vi "Process Imported Data.vi"(8 "error in (no error)":errorcluster, 10 "Raw File Data":string, 11 "State Data in":T1={"Raw File Data"="", "Deduplicated String Array"=[], "1-Entries"=[], "2-Entries"=[], "3-Entries"=[], "Bounds"={"M-Min"=0, "M-Max"=1023, "S-Min"=0, "S-Max"=1023}, "Matched ADC Values - Nearest"=[], "Match Entry Indices - Nearest"=[], "Filtered 1-Entries"=[], "Filtered 2-Entries"=[], "Filtered 3-Entries"=[], "Total Duration"=0.0, "Matched ADC Values - Largest"=[], "Match Entry Indices - Largest"=[]}) -> (0 "error out":errorcluster, 3 "State Data out":T1={"Raw File Data"="", "Deduplicated String Array"=[], "1-Entries"=[], "2-Entries"=[], "3-Entries"=[], "Bounds"={"M-Min"=0, "M-Max"=1023, "S-Min"=0, "S-Max"=1023}, "Matched ADC Values - Nearest"=[], "Match Entry Indices - Nearest"=[], "Filtered 1-Entries"=[], "Filtered 2-Entries"=[], "Filtered 3-Entries"=[], "Total Duration"=0.0, "Matched ADC Values - Largest"=[], "Match Entry Indices - Largest"=[]})   [LabVIEW 2019, in "Muon Data Post-Processing.lvlib"]
uses:
  Muon Data Post-Processing.lvlib
  State Data.ctl
  File Entry.ctl
  ADC Bounds.ctl
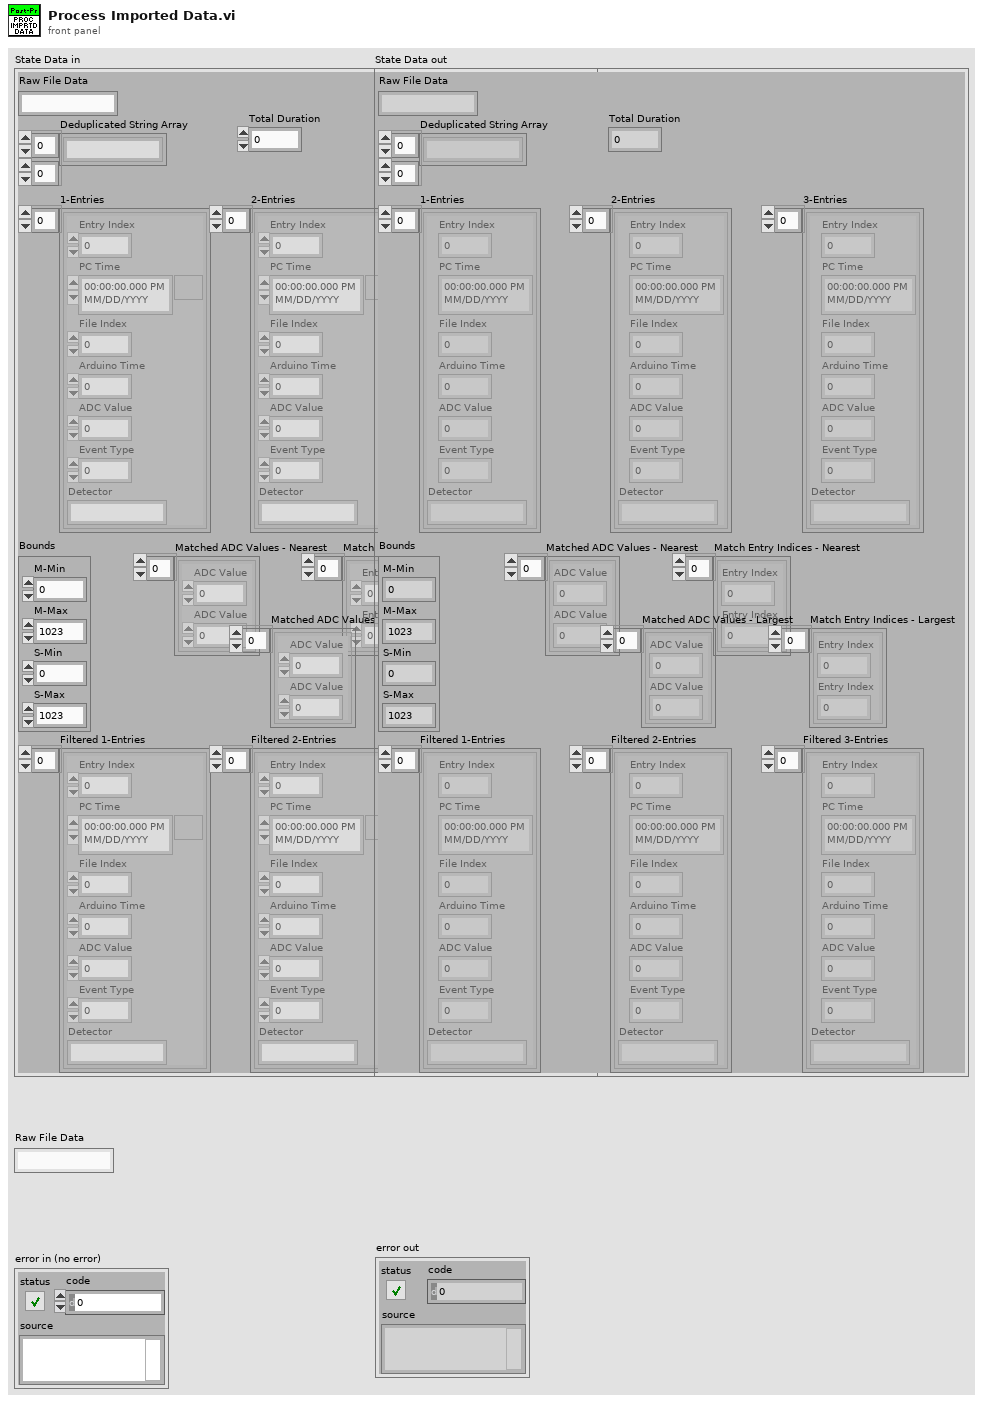
[diagram p1: front panel]
types:
  T1 = typedef "Muon Data Post-Processing.lvlib/State Data.ctl" = cluster{"Raw File Data":string, "Deduplicated String Array":string[][], "1-Entries":T2[], "2-Entries":T2[], "3-Entries":T2[], "Bounds":T3, "Matched ADC Values - Nearest":cluster{"ADC Value":i32, "ADC Value":i32}[], "Match Entry Indices - Nearest":cluster{"Entry Index":i32, "Entry Index":i32}[], "Filtered 1-Entries":T2[], "Filtered 2-Entries":T2[], "Filtered 3-Entries":T2[], "Total Duration":dbl, "Matched ADC Values - Largest":cluster{"ADC Value":i32, "ADC Value":i32}[], "Match Entry Indices - Largest":cluster{"Entry Index":i32, "Entry Index":i32}[]}
  T2 = typedef "Muon Data Post-Processing.lvlib/File Entry.ctl" = cluster{"Entry Index":i32, "PC Time":timestamp, "File Index":i32, "Arduino Time":i32, "ADC Value":i32, "Event Type":i32, "Detector":string}
  T3 = typedef "Muon Data Post-Processing.lvlib/ADC Bounds.ctl" = cluster{"M-Min":u16, "M-Max":u16, "S-Min":u16, "S-Max":u16}
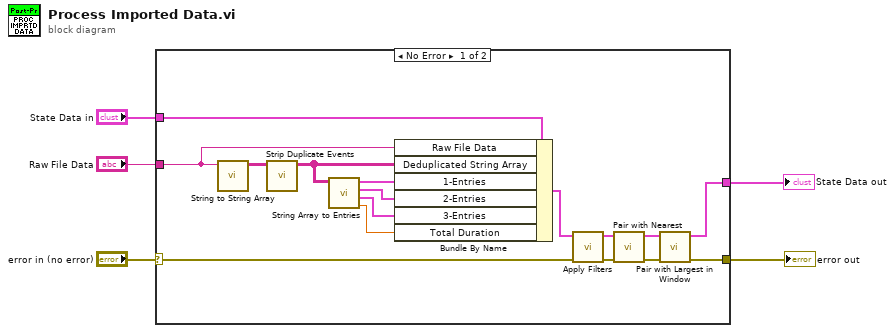
[diagram p0: block diagram]
diagram:
  n1 = case shown="No Error" "error in (no error)" {
    selector: "error in (no error)" -> [w18 w23]
    tunnel: "State Data in" -> [w20 w22]
    tunnel: "Raw File Data" -> [w19 _]
    tunnel: [w6 w22] -> w3
    tunnel: [w8 w23] -> w1
    frame No Error {
      n2 = call "String to String Array.vi"("String"=w19) -> ("Array"=w21:string[][])  [unwired: 10 in]
      n3 = call "Strip Duplicate Events.vi"("Array in"=w21) -> ("Array out"=w17:string[][])  [unwired: 8 in, 2 out]
      n4 = call "String Array to Entries.vi"("String Array in"=w17) -> ("Total Duration"=w9:dbl, "3-Entries"=w14:T2[], "2-Entries"=w15:T2[], "1-Entries"=w16:T2[])  [unwired: 7 in]
      n5 = Bundle By Name(cluster=w20, "Raw File Data"=w19, "Deduplicated String Array"=w17, "1-Entries"=w16, "2-Entries"=w15, "3-Entries"=w14, "Total Duration"=w9) -> (w11:T1)
      n6 = call "Apply Filters.vi"("error in (no error)"=w18, "State in"=w11) -> ("error out"=w12:errorcluster, "State out"=w10:T1)  [unwired: 8 in]
      n7 = call "Pair with Nearest.vi"("error in (no error)"=w12, "State in"=w10) -> ("error out"=w13:errorcluster, "State out"=w7:T1)  [unwired: 8 in]
      n8 = call "Pair with Largest in Window.vi"("error in (no error)"=w13, "State in"=w7) -> ("error out"=w8:errorcluster, "State out"=w6:T1)  [unwired: 8 in]
    }
    frame Error {
    }
  }
  "error out" <- w1
  "State Data out" <- w3
